vi "SIM_FrameProperties.vi"() -> (0 "data":dbl[][](array[numeric]), 1 "Surf Loc (m)":dbl, 2 "Size (m)":cluster{"Width":sgl, "Height":sgl}, 3 "Center coordinates (m)":cluster{"Xc":sgl, "Yc":sgl})   [LabVIEW 2017]
uses:
  <vilib>/Utility/file.llb/Read Delimited Spreadsheet (DBL).vi
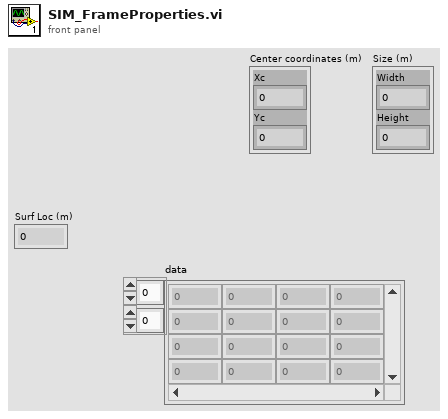
[diagram p1: front panel]
types:
  T1 = cluster{"[0]":dbl, "[1]":dbl, "[2]":dbl, "[3]":dbl, "[4]":dbl, "[5]":dbl, "[6]":dbl, "[7]":dbl, "[8]":dbl}
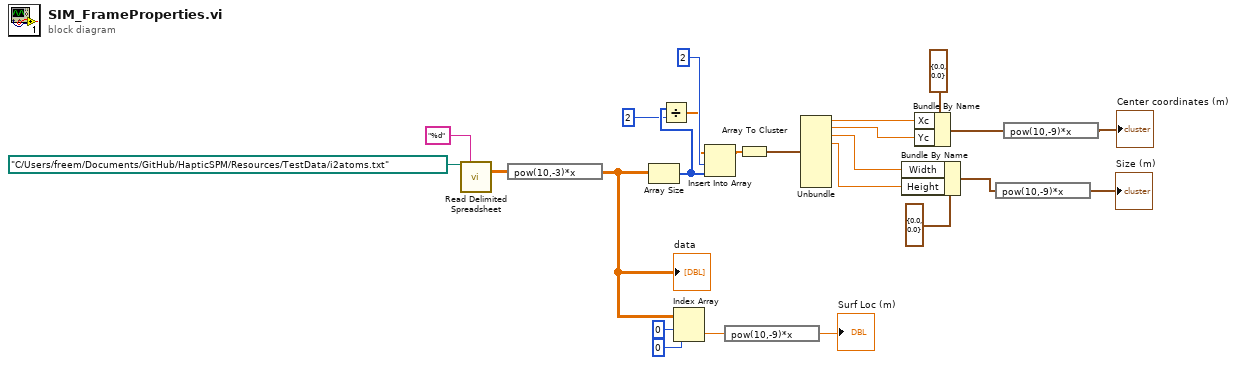
[diagram p0: block diagram]
diagram:
  n1 = call-poly <vilib>:"Read Delimited Spreadsheet.vi"("file path (dialog if empty)"=path "C:/Users/freem/Documents/GitHub/HapticSPM/Resources/TestData/i2atoms.txt", "format (%.3f)"="%d") -> ("all rows"=w16:dbl[][])  [unwired: 8 in, 5 out]
  n2 = expression code="pow(10,-3)*x"(w16) -> (w15:dbl[][])
  "data" <- w15
  n3 = Array Size(array=w15) -> (size(s)=w9:i32[])
  n4 = Divide(x=w9, y=2) -> (x/y=w10:dbl[])
  n5 = Index Array(array=w15, index (row)=0, index (col)=0 ("disabled index (col)")) -> (element=w13:dbl)
  n6 = Insert Into Array(array=w10, index=2, new element=w9) -> (w22:dbl[])
  n7 = expression code="pow(10,-9)*x"(w13) -> (→"Surf Loc (m)":dbl)
  n8 = Array To Cluster(array=w22) -> (cluster=w21:T1)
  n9 = Unbundle(w21) -> ("[0]"=w20:dbl, "[1]"=w19:dbl, "[2]"=w2:dbl, "[3]"=w1:dbl)  [unwired: 5 out]
  n10 = Bundle By Name(cluster=cluster{"Width":sgl, "Height":sgl} {"Width"=0.0, "Height"=0.0} ("Size (m)"), "Width"=w2, "Height"=w1) -> (w4:cluster{"Width":sgl, "Height":sgl})
  n11 = Bundle By Name(cluster=cluster{"Xc":sgl, "Yc":sgl} {"Xc"=0.0, "Yc"=0.0} ("Center coordinates (m)"), "Xc"=w20, "Yc"=w19) -> (w12:cluster{"Xc":sgl, "Yc":sgl})
  n12 = expression code="pow(10,-9)*x"(w4) -> (→"Size (m)":cluster{"Width":sgl, "Height":sgl})
  n13 = expression code="pow(10,-9)*x"(w12) -> (→"Center coordinates (m)":cluster{"Xc":sgl, "Yc":sgl})
